vi "Disconnect_Variable_Typedefs.vi"(8 "error in (no error)":errorcluster, 11 "library reference in":refnum<vi>) -> (0 "error out":errorcluster, 3 "library reference out":refnum<vi>)   [LabVIEW 2020, in "AB_Source_Library.lvclass"]
uses:
  <vilib>/AppBuilder/AB_Classes/Source/Library/AB_Source_Library.lvclass
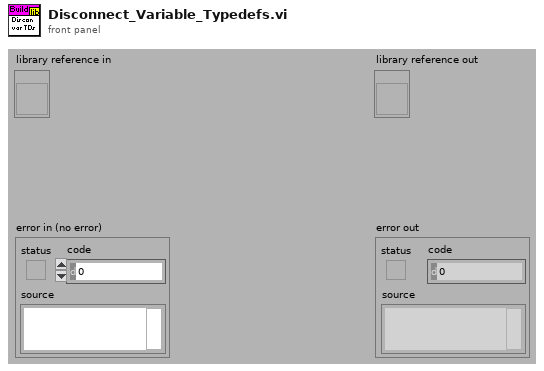
[diagram p1: front panel]
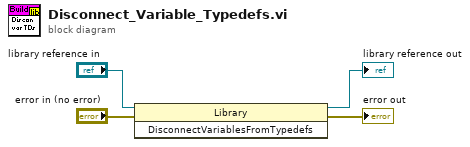
[diagram p0: block diagram]
diagram:
  n1 = invoke class="Library" method="DisconnectVariablesFromTypedefs"(reference="library reference in", error in="error in (no error)") -> (reference out=→"library reference out":refnum<vi>, error out=→"error out":errorcluster)  [unwired: 1 in, 1 out]
